vi "SubscribeEvent.vi"(0 "device name":string, 1 "attribute name":string, 2 "evt type":i16, 3 "error in":errorcluster, 4 "Tango Atttibute Value Event Refnum":refnum<event-registration>) -> (5 "error out":errorcluster)   [LabVIEW 2014, in "tango.lvlib"]
uses:
  tango.lvlib
  tango_binding.so
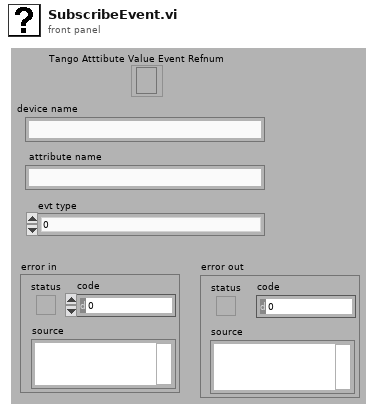
[diagram p1: front panel]
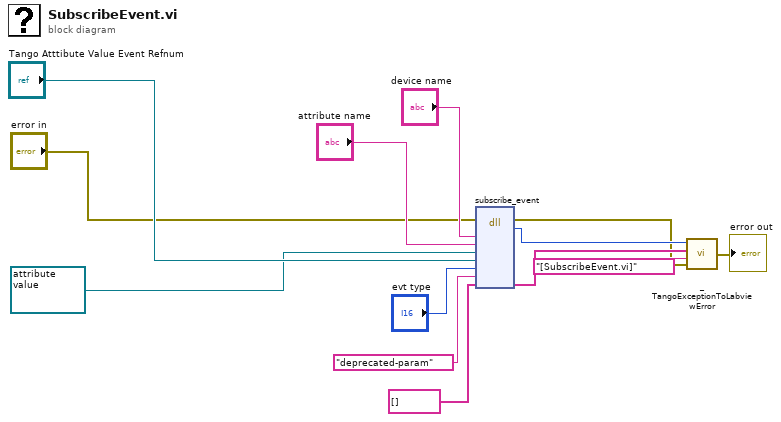
[diagram p0: block diagram]
diagram:
  n1 = dll-call lib="tango_binding.*" fn="subscribe_event"(error in="error in", "dev_name"="device name", "attr_name"="attribute name", "evt_refnum_dll"=refnum<user-event> refnum, "evt_refnum_lv"="Tango Atttibute Value Event Refnum", "evt_type"="evt type", "evt_filters"="deprecated-param", "error_stack_"=string[] [] ("subscribe error stack")) -> (error out=w4:errorcluster, "return type"=w7:i32, "error_stack_"=w6:string[])  [unwired: 8 in, 1 out]
  n2 = call "_TangoExceptionToLabviewError.vi"("error in"=w4, "location"="[SubscribeEvent.vi]", "error stack"=w6, "error code"=w7) -> ("error out"=→"error out":errorcluster)
